vi "OTP - Generate Keys File.vi"(9 "Key Length":i32=10, 10 "Lines":i32=100000, 11 "File Path":path) -> ()   [LabVIEW 2013]
panel:
  out "spreadsheet string":string
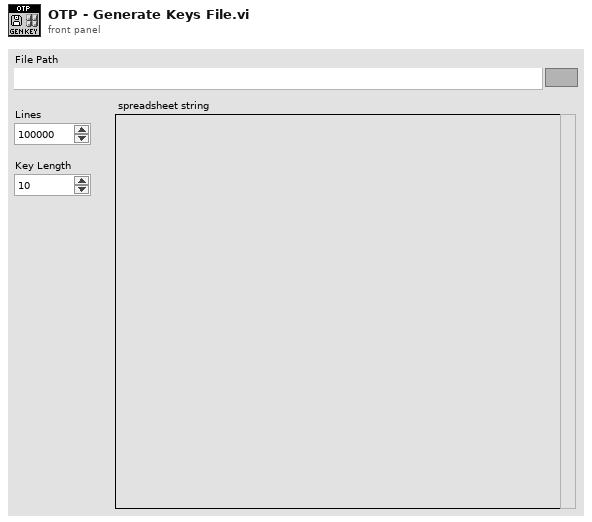
[diagram p1: front panel]
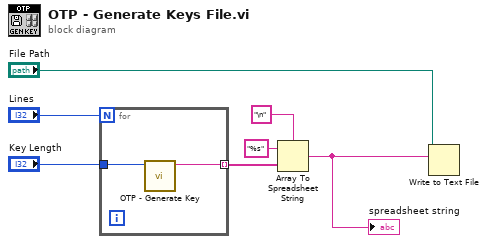
[diagram p0: block diagram]
diagram:
  n1 = for {
    N: "Lines" -> [_]
    tunnel: "Key Length" -> [w9]
    tunnel: [w8] -> w5 mode=indexing
    n2 = call "OTP - Generate Key.vi"("Length"=w9) -> ("key (Private)"=w8:string)  [unwired: 10 in]
  }
  n3 = Array To Spreadsheet String(delimiter (Tab)="\n", array=w5, 3:"%s" ("format string")) -> (spreadsheet string=w2:string)
  "spreadsheet string" <- w2
  n4 = Write to Text File(file (use dialog)="File Path", text=w2) -> ()  [unwired: 2 in, 3 out]
